vi "Set Color.vi"(8 "error in (no error)":errorcluster, 10 "Color Message.lvclass":refnum<class "Color Message.lvclass">, 11 "[V]Waveform Display in":refnum<class "[V]Waveform Display.lvclass">) -> (0 "error out":errorcluster, 3 "[V]Waveform Display out":refnum<class "[V]Waveform Display.lvclass">)   [LabVIEW 2020, in "[V]Waveform Display.lvlib" / "[V]Waveform Display.lvclass"]
uses:
  [V]Waveform Display.lvclass
  Color Interface/Color/Color Message.lvclass
  Depden On/Abstruct View/Abstruct View/Abstruct View.lvclass/Abstruct View.ctl
  Color Interface/Color/Color Message.lvclass/Color Message.ctl
  Color Interface/Color/Accessors/Read BG Color.vi
  Depden On/Abstruct View/Abstruct View/Data Accessors/Read Core VI.vi
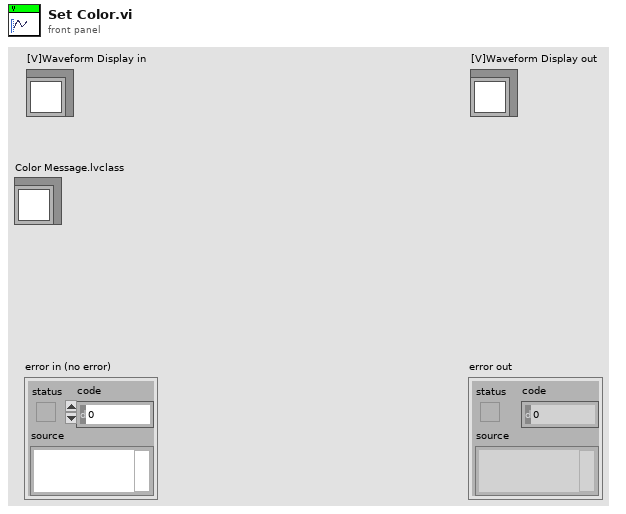
[diagram p1: front panel]
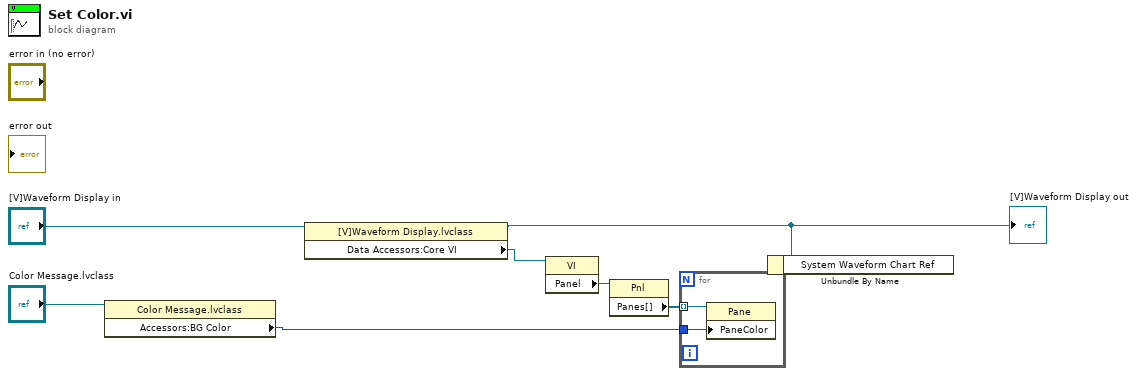
[diagram p0: block diagram]
diagram:
  n1 = property class="Color Message.lvclass"(reference="Color Message.lvclass") -> ("Accessors:BG Color"=w1:u32)  [unwired: 1 in, 2 out]
  n2 = property class="[V]Waveform Display.lvclass"(reference="[V]Waveform Display in") -> (reference out=w2:refnum<class "[V]Waveform Display.lvclass">, "Data Accessors:Core VI"=w5:refnum<vi>)  [unwired: 1 in, 1 out]
  "[V]Waveform Display out" <- w2
  n3 = property class="VI"(reference=w5) -> ("Panel"=w4:refnum<vi>)  [unwired: 1 in, 2 out]
  n4 = property class="Pnl"(reference=w4) -> ("Panes[]"=w3:refnum<vi>[])  [unwired: 1 in, 2 out]
  n5 = for {
    tunnel: w3 -> [w9] mode=indexing
    tunnel: w1 -> [w8]
    n6 = property class="Pane"(reference=w9, "PaneColor"=w8) -> ()  [unwired: 1 in, 2 out]
  }
  n7 = Unbundle By Name(w2) -> ()  [unwired: 1 out]
